vi "Panel.vi"(5 "Show Event":refnum<user-event>, 7 "Stop Event":refnum<user-event>, 9 "Label":string, 10 "Panel":refnum<class "Panel.lvclass">) -> ()   [LabVIEW 2020, in "1. Basic Panels.lvlib"]
doc: "This is a basic panel. \n\nIt doesn't know what type of panel it is until runtime, this means that whoever launches this VI can define what type of panel it will be.\n----\nCopyright: MGI 2016\nAuthor: Derek Trepanier"
uses:
  1. Basic Panels.lvlib
  <vilib>/MGI/Panel Manager/Panel/Panel/Panel.lvclass
panel:
  out "Label Out":string
  in  "Show Dialog":bool
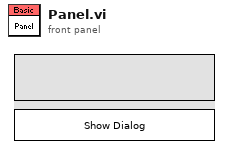
[diagram p1: front panel]
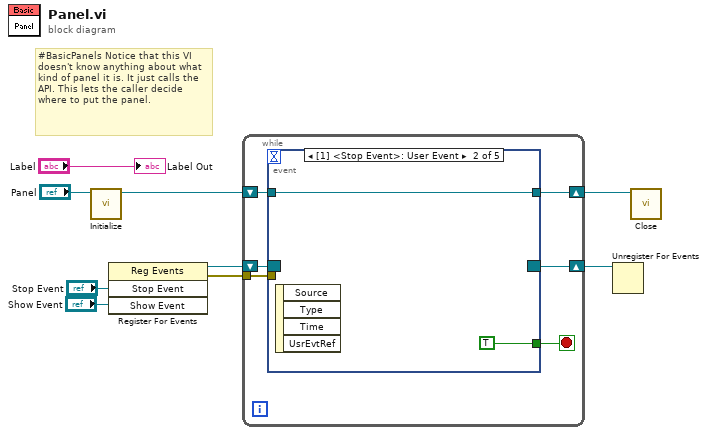
[diagram p0: block diagram]
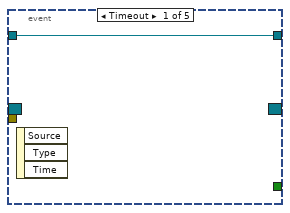
[diagram p2: hidden frame]
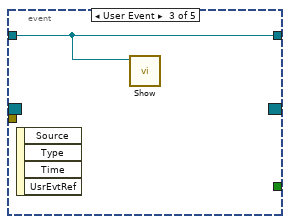
[diagram p3: hidden frame]
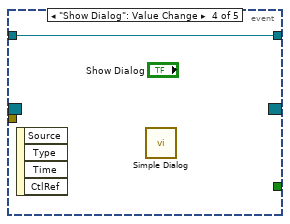
[diagram p4: hidden frame]
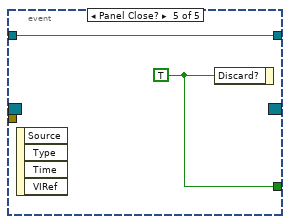
[diagram p5: hidden frame]
diagram:
  # "#BasicPanels Notice that this VI doesn't know anything about what kind of panel it is. It just calls the API. This lets the caller decide where to put the panel."
  n1 = call <vilib>:"Initialize.vi"("Panel In"="Panel") -> ("Panel Out"=w5:refnum<class "Panel.lvclass">)  [unwired: 8 in, 2 out]
  n2 = register-events("Stop Event", "Show Event") -> (reference out=w6:refnum<event-registration>, error out=w1:errorcluster)  [unwired: 2 in]
  n3 = while {
    tunnel: w1 -> [w11]
    shift-right: [w12] -> w3
    shift-left: w6 -> [w15]
    shift-right: [w13] -> w4
    shift-left: w5 -> [w14]
    stop <- w10 stop-if-true
    n4 = event shown="[1] <Stop Event>: User Event" {
      selector: w15 -> [_ _ _ _ _]
      dyn-events: [_ _ _ _ _] -> w12
      timeout: _ -> [_ _ _ _ _]
      tunnel: w14 -> [w16 w18 w19 w20 w22]
      tunnel: [w16 w18 w19 w20 w22] -> w13
      tunnel: w11 -> [_ _ _ _ _]
      tunnel: [_ TRUE _ _ w21] -> w10
      event Timeout {
        n5 = event-data() -> ()  [unwired: 1 in, 3 out]
      }
      event User Event {
        n6 = event-data() -> ()  [unwired: 1 in, 4 out]
      }
      event User Event {
        n7 = event-data() -> ()  [unwired: 1 in, 4 out]
        n8 = call <vilib>:"Show.vi"("Panel in"=w19) -> ()  [unwired: 10 in, 1 out]
      }
      event "Show Dialog": Value Change {
        n9 = event-data() -> ()  [unwired: 1 in, 4 out]
        n10 = call "Simple Dialog.vi"() -> ()  [unwired: 12 in]
      }
      event Panel Close? {
        w21 = TRUE ("Discard?")
        n11 = event-data() -> ()  [unwired: 1 in, 4 out]
        n12 = event-data("Discard?"=w21) -> ()  [unwired: 1 in, 1 out]
      }
    }
  }
  n13 = Unregister For Events(event registration refnum=w3) -> ()  [unwired: 1 in, 1 out]
  n14 = call-dynamic "Close.vi"("Panel In"=w4) -> ()  [unwired: 10 in, 1 out]
  "Label Out" <- "Label"
